vi "Redirect.vi"(6 "LabVIEW Web Service Request":refnum<class "Web Request.lvclass">) -> (1 "query string":string)   [LabVIEW 2019]
uses:
  <vilib>/wsapi/Web Request.lvclass
  Useful OAuth VIs/globals.vi
  Useful OAuth VIs/Useful OAuth VIs.lvlib
  Useful HTTP VIs/Useful HTTP VIs.lvlib
panel:
  # "Each additional control wired to the connector pane will be available as an input in the URL. To include an indicator in terminal-mode output (the default setting), it must also be wired to the connector pane."
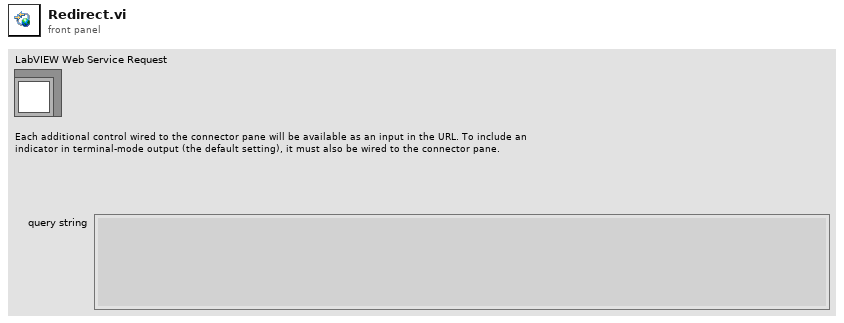
[diagram p1: front panel]
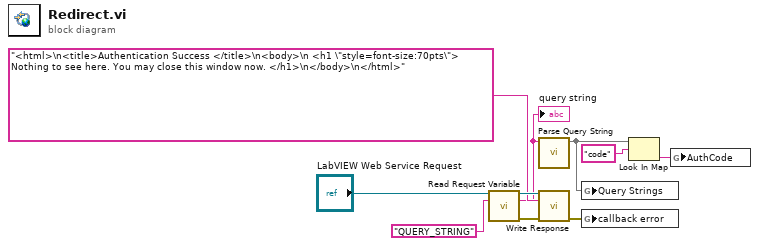
[diagram p0: block diagram]
diagram:
  n1 = call <vilib>:"Read Request Variable.vi"("LabVIEW Web Service Request"="LabVIEW Web Service Request", "variable name"="QUERY_STRING") -> ("LabVIEW Web Service Request out"=w8:refnum<class "Web Request.lvclass">, "value"=w5:string, "error out"=w6:errorcluster)  [unwired: 11 in]
  "query string" <- w5
  n2 = call "Parse Query String.vi"("query string"=w5) -> ("Map"=w3:map{string, string})  [unwired: 10 in]
  n3 = call <vilib>:"Write Response.vi"("LabVIEW Web Service Request"=w8, "response string"="<html>\n<title>Authentication Success </title>\n<body>\n <h1 \"style=font-size:70pts\"> Nothing to see here. You may close this window now. </h1>\n</body>\n</html>", "error in (no error)"=w6) -> ("error out"=w4:errorcluster)  [unwired: 11 in, 1 out]
  n4 = global write "globals.vi" "Query Strings"(w3) -> ()
  n5 = global write "globals.vi" "callback error"(w4) -> ()
  n6 = Look In Map(map=w3, key="code") -> (value=w1:string)  [unwired: 1 in, 1 out]
  n7 = global write "globals.vi" "AuthCode"(w1) -> ()
